vi "PH_Tektronix_7000.Evt Call Set Trigger Configuration.vi"(0 "i ref in":refnum<vi>, 1 "Instance":string="N/A", 2 "Trigger Configuration":T1 {"Trigger Mode" items=["Normal", "Auto"]; "Coupling" items=["DC", "AC", "Hf Reject", "Lf Reject", "Noise Rej", "Atrigger"]; "Slope" items=["Rise", "Fall", "Either"]; "Source" items=["Channel1"=0, "Channel2"=1, "Channel3"=2, "Channel4"=3, "Aux"=12, "Line"=13]}, 5 "error in (no error)":errorcluster) -> (14 "i ref out":refnum<vi>, 19 "error out":errorcluster)   [LabVIEW 2014, in "PH_Tektronix_7000.lvlib"]
doc: "This VI calls sets a simple call."
uses:
  PH_Tektronix_7000.lvlib
  PH_Tektronix_7000.Trigger Config.ctl
  CS_Core/CSSystem/CoreLib/CoreLib.short 2 byte array.vi
  CS_Core/CSSystem/CoreLib/CoreLib.double 2 byte array.vi
  CS_Core/CSSystem/CoreLib/CoreLib.lvlib
  CS_Core/BaseProcess/BaseProcess.lvlib
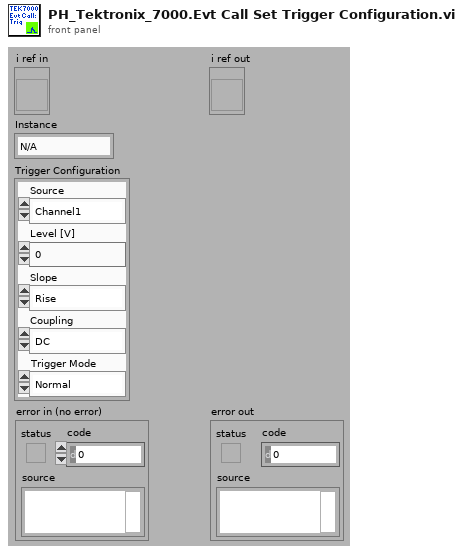
[diagram p1: front panel]
types:
  T1 = typedef "PH_Tektronix_7000.lvlib/PH_Tektronix_7000.Trigger Config.ctl" = cluster{"Source":u16, "Level [V]":dbl, "Slope":u16, "Coupling":u16, "Trigger Mode":u16}
  T2 = typedef "CoreDefs.rawDataType.ctl" = i8[]
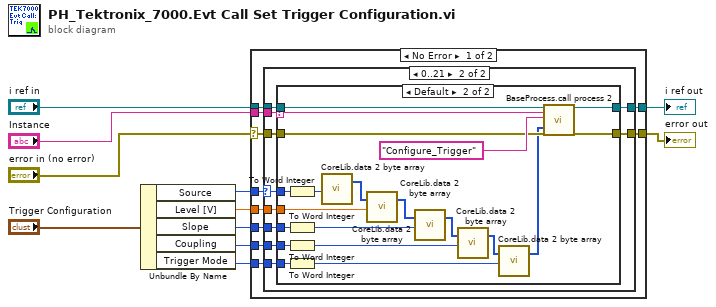
[diagram p0: block diagram]
diagram:
  n1 = Unbundle By Name("Trigger Configuration") -> ("Source"=w5:u16, "Level [V]"=w4:dbl, "Slope"=w3:u16, "Coupling"=w2:u16, "Trigger Mode"=w1:u16)
  n2 = case shown="No Error" "error in (no error)" {
    selector: "error in (no error)" -> [w17 w56]
    tunnel: [w21 w57] -> w11
    tunnel: [w20 w56] -> w10
    tunnel: "i ref in" -> [w19 w57]
    tunnel: w5 -> [w16 _]
    tunnel: "Instance" -> [w18 _]
    tunnel: w4 -> [w15 _]
    tunnel: w3 -> [w14 _]
    tunnel: w2 -> [w13 _]
    tunnel: w1 -> [w12 _]
    frame No Error {
      n3 = case shown="0..21" w16 {
        selector: w16 -> [_ w28]
        tunnel: [w23 w33] -> w21
        tunnel: [w22 w32] -> w20
        tunnel: w19 -> [w23 w31]
        tunnel: w18 -> [_ w30]
        tunnel: w17 -> [w22 w29]
        tunnel: w15 -> [_ w27]
        tunnel: w14 -> [_ w26]
        tunnel: w13 -> [_ w25]
        tunnel: w12 -> [_ w24]
        frame Default {
        }
        frame 0..21 {
          n4 = case shown="Default" w30 {
            selector: w30 -> [_ w50]
            tunnel: [w34 w54] -> w33
            tunnel: [w35 w53] -> w32
            tunnel: w31 -> [w34 w52]
            tunnel: w29 -> [w35 w51]
            tunnel: w28 -> [_ w49]
            tunnel: w27 -> [_ w48]
            tunnel: w26 -> [_ w46]
            tunnel: w25 -> [_ w44]
            tunnel: w24 -> [_ w37]
            frame "N/A" {
            }
            frame Default {
              n5 = To Word Integer(number=w49) -> (16bit integer=w42:i16)
              n6 = To Word Integer(number=w46) -> (16bit integer=w41:i16)
              n7 = To Word Integer(number=w44) -> (16bit integer=w40:i16)
              n8 = To Word Integer(number=w37) -> (16bit integer=w36:i16)
              n9 = call-poly "CoreLib.data 2 byte array.vi"("i16"=w42) -> ("byteArray out"=w47:T2)  [unwired: 18 in]
              n10 = call-poly "CoreLib.data 2 byte array.vi"("byteArray"=w47, "f64"=w48) -> ("byteArray out"=w45:T2)  [unwired: 17 in]
              n11 = call-poly "CoreLib.data 2 byte array.vi"("byteArray"=w45, "i16"=w41) -> ("byteArray out"=w43:T2)  [unwired: 17 in]
              n12 = call-poly "CoreLib.data 2 byte array.vi"("byteArray"=w43, "i16"=w40) -> ("byteArray out"=w39:T2)  [unwired: 17 in]
              n13 = call-poly "CoreLib.data 2 byte array.vi"("byteArray"=w39, "i16"=w36) -> ("byteArray out"=w38:T2)  [unwired: 17 in]
              n14 = call "BaseProcess.call process 2.vi"("i ref in"=w52, "Object"=w50, "Selector"="Configure_Trigger", "Data"=w38, "error in (no error)"=w51) -> ("i ref out"=w54:refnum<vi>, "error out"=w53:errorcluster)  [unwired: 13 in]
            }
          }
        }
      }
    }
    frame Error {
    }
  }
  "i ref out" <- w11
  "error out" <- w10
